vi "String to Variant.vi"(8 "error in (no error)":errorcluster, 10 "String":string, 11 "Timestamp Value in":refnum<class "Timestamp Value.lvclass">) -> (0 "error out":errorcluster, 2 "Variant":variant, 3 "Timestamp Value out":refnum<class "Timestamp Value.lvclass">)   [LabVIEW 2020, in "Composed Columns.lvlib" / "Timestamp Value.lvclass"]
uses:
  Timestamp Value.lvclass
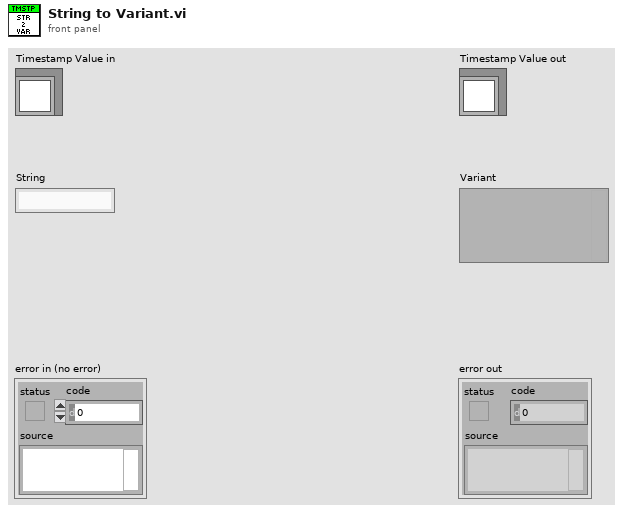
[diagram p1: front panel]
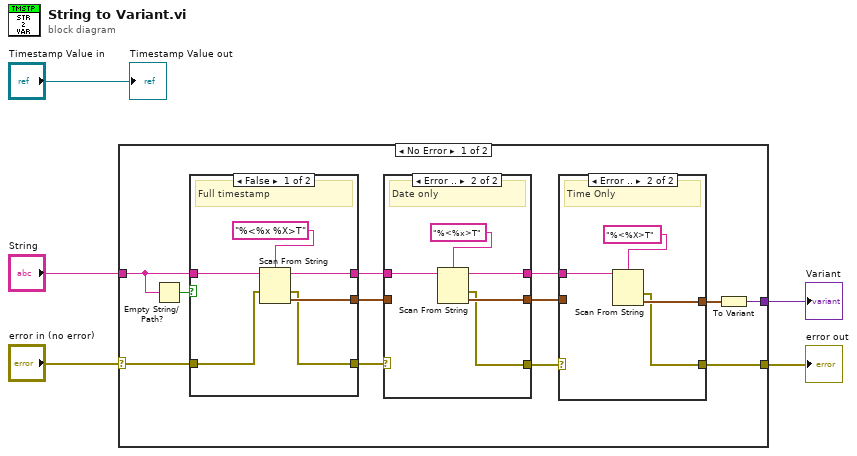
[diagram p0: block diagram]
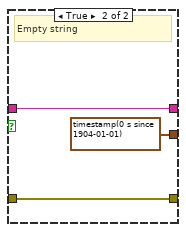
[diagram p4: hidden frame]
diagram:
  n1 = case shown="No Error" "error in (no error)" {
    selector: "error in (no error)" -> [w17 w41]
    tunnel: "String" -> [w15 _]
    tunnel: [w8 w41] -> w3
    tunnel: [w6 _] -> w2
    frame No Error {
      n2 = Empty String/Path?(string/path=w15) -> (empty?=w16:bool)
      n3 = case shown="False" w16 {
        tunnel: w15 -> [w36 w38]
        tunnel: [w35 timestamp(0 s since 1904-01-01)] -> w12
        tunnel: w17 -> [w34 w39]
        tunnel: [w33 w39] -> w14
        tunnel: [w32 w38] -> w13
        frame False {
          # "Full timestamp"
          n4 = Scan From String(format string="%<%x %X>T", input string=w36, error in=w34) -> (remaining string=w32:string, error out=w33:errorcluster, output 1=w35:timestamp)  [unwired: 2 in, 1 out]
        }
        frame True {
          # "Empty string"
        }
      }
      n5 = case shown="Error .." w14 {
        selector: w14 -> [w26 _]
        tunnel: [w25 w30] -> w10
        tunnel: [w26 w29] -> w11
        tunnel: w13 -> [w24 w28]
        tunnel: w12 -> [w25 _]
        tunnel: [w24 w27] -> w9
        frame No Error {
          # "Already parsed"
        }
        frame Error {
          # "Date only"
          n6 = Scan From String(format string="%<%x>T", input string=w28) -> (remaining string=w27:string, error out=w29:errorcluster, output 1=w30:timestamp)  [unwired: 3 in, 1 out]
        }
      }
      n7 = case shown="Error .." w11 {
        selector: w11 -> [w19 _]
        tunnel: [w18 w22] -> w7
        tunnel: [w19 w21] -> w8
        tunnel: w9 -> [_ w20]
        tunnel: w10 -> [w18 _]
        frame No Error {
          # "Already Parsed"
        }
        frame Error {
          # "Time Only"
          n8 = Scan From String(format string="%<%X>T", input string=w20) -> (error out=w21:errorcluster, output 1=w22:timestamp)  [unwired: 3 in, 2 out]
        }
      }
      n9 = To Variant(anything=w7) -> (Variant=w6:variant)
    }
    frame Error {
    }
  }
  "error out" <- w3
  "Variant" <- w2
  "Timestamp Value out" <- "Timestamp Value in"
